vi "Get Parameter List.vi"(8 "error in":errorcluster, 11 "Detector in":refnum<class "PID.lvclass">) -> (0 "error out":errorcluster, 1 "values":variant[](array[variant]), 2 "names":string[](array[string]), 3 "Detector out":refnum<class "PID.lvclass">)   [LabVIEW 2011, in "PID.lvclass"]
doc: "Fetch the parameters associated with the last spectral data acquistion."
uses:
  PID.lvclass
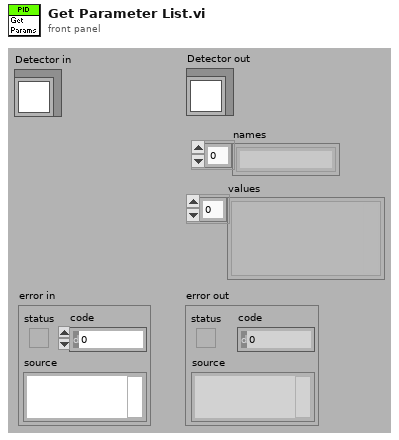
[diagram p1: front panel]
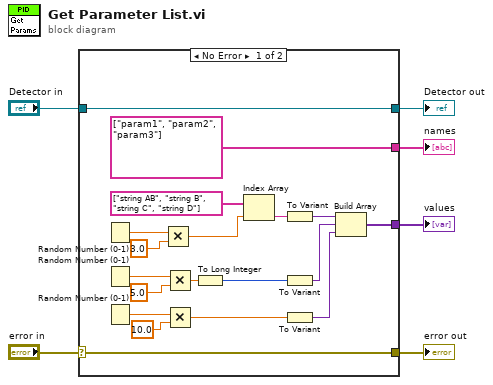
[diagram p0: block diagram]
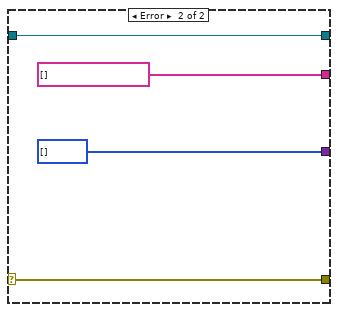
[diagram p2: hidden frame]
diagram:
  n1 = case shown="No Error" "error in" {
    selector: "error in" -> [w24 w29]
    tunnel: [w24 w29] -> w5
    tunnel: [w25 w28] -> w3
    tunnel: "Detector in" -> [w25 w28]
    tunnel: [string[] ["param1", "param2", "param3"] ("names") string[] [] ("names")] -> w2
    tunnel: [w20 i16[] [] ("values")] -> w1
    frame No Error {
      n2 = Random Number (0-1)() -> (number: 0 to 1=w12:dbl)
      n3 = Random Number (0-1)() -> (number: 0 to 1=w19:dbl)
      n4 = Random Number (0-1)() -> (number: 0 to 1=w16:dbl)
      n5 = Multiply(x=w12, y=3.0) -> (x*y=w9:dbl)
      n6 = Multiply(x=w19, y=5.0) -> (x*y=w14:dbl)
      n7 = Multiply(x=w16, y=10.0) -> (x*y=w15:dbl)
      n8 = To Long Integer(number=w14) -> (32bit integer=w13:i32)
      n9 = Index Array(array=string[] ["string AB", "string B", "string C", "string D"] ("names"), index=w9) -> (element=w8:string)
      n10 = To Variant(anything=w8) -> (Variant=w22:variant)
      n11 = To Variant(anything=w13) -> (Variant=w21:variant)
      n12 = To Variant(anything=w15) -> (Variant=w7:variant)
      n13 = Build Array(w22, w21, w7) -> (w20:variant[])
    }
    frame Error {
    }
  }
  "error out" <- w5
  "Detector out" <- w3
  "names" <- w2
  "values" <- w1
